vi "lowpass_derivative.vi"(9 "sigma_time":dbl=10.0 format="%#_13g", 10 "sampling frequency":dbl=0.1, 11 "X":dbl[](array[numeric])) -> (3 "dX":dbl[](array[numeric]))   [LabVIEW 2017]
uses:
  <vilib>/Analysis/2dsp.llb/1D Convolution (DBL).vi
  <vilib>/Analysis/1siggen.llb/General Gaussian Monopulse.vi
  <vilib>/Analysis/NI_AALBase.lvlib
  <vilib>/Analysis/NI_AALPro.lvlib
panel:
  out "input size":i32
  out "kernel size":i32
  out "Y":dbl[](graph)
  out "graph of dX":dbl[](graph)
  out "conv":dbl[](graph)
  out "X":dbl[](graph)
  out "pad size":i32
  out "conv size":i32
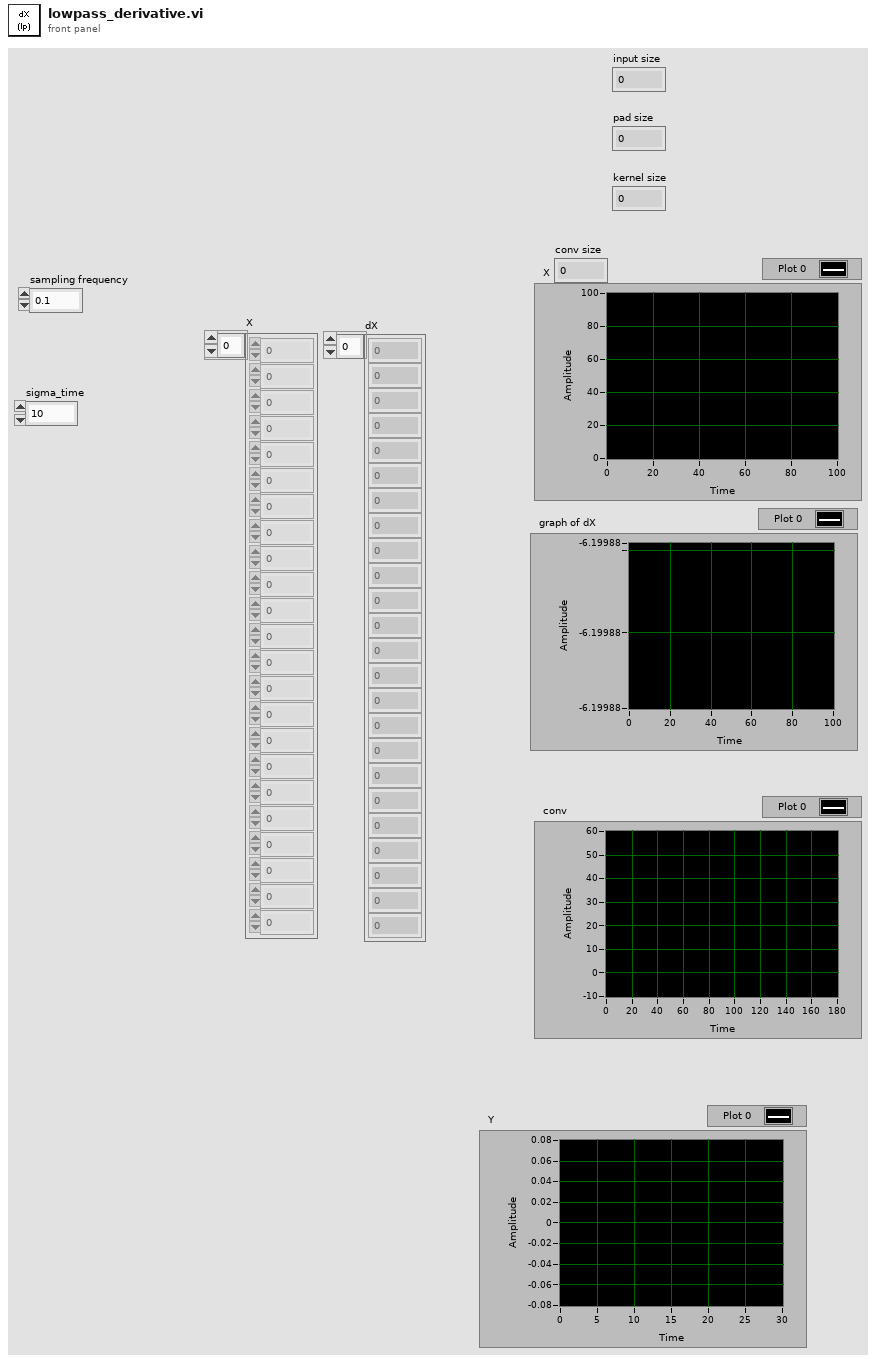
[diagram p1: front panel]
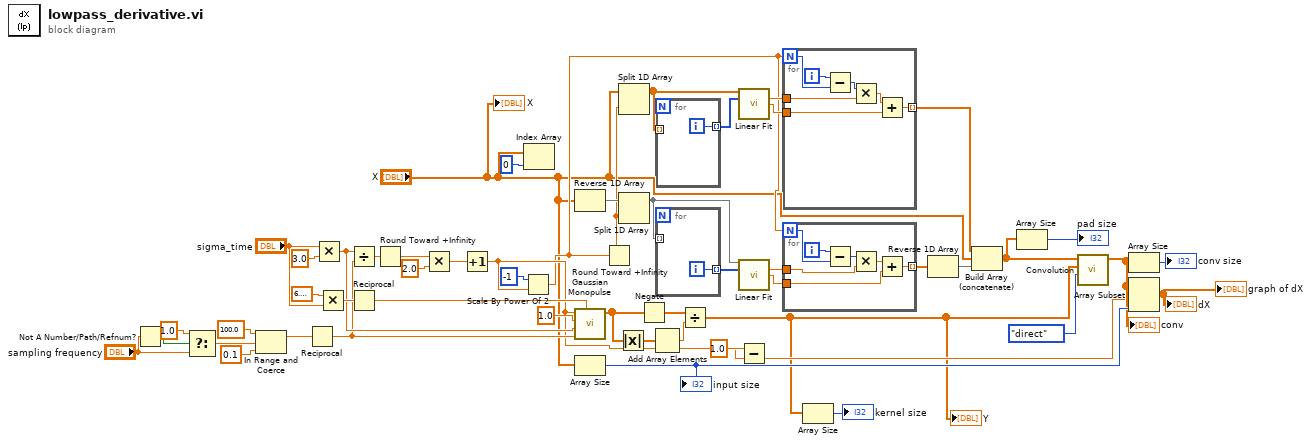
[diagram p0: block diagram]
diagram:
  n1 = Not A Number/Path/Refnum?(number/path/refnum="sampling frequency") -> (NaN/Path/Refnum?=w35:bool)
  n2 = Select(t=1.0, s=w35, f="sampling frequency") -> (s? t:f=w32:dbl)
  n3 = In Range and Coerce(upper limit=100.0, x=w32, lower limit=0.1) -> (coerced(x)=w38:dbl)  [unwired: 1 out]
  n4 = Reciprocal(x=w38) -> (1/x=w26:dbl)
  n5 = Multiply(x="sigma_time", y=3.0) -> (x*y=w47:dbl)
  n6 = Multiply(x=6.283185307179586, y="sigma_time") -> (x*y=w50:dbl)
  n7 = Divide(x=w47, y=w26) -> (x/y=w46:dbl)
  n8 = Reciprocal(x=w50) -> (1/x=w27:dbl)
  n9 = Round Toward +Infinity(x=w46) -> (ceil(x): smallest int >= x=w45:dbl)
  n10 = Multiply(x=w45, y=2.0) -> (x*y=w43:dbl)
  n11 = Increment(x=w43) -> (x+1=w8:dbl)
  n12 = Scale By Power Of 2(n=i16 -1, x=w8) -> (x*2^n=w3:dbl)
  n13 = Index Array(array="X", index=0) -> ()  [unwired: 1 out]
  n14 = Reverse 1D Array(array="X") -> (reversed array=w19:dbl[])
  n15 = call <vilib>:"Gaussian Monopulse.vi"("center frequency (Hz)"=w27, "delta t (s)"=w26, "delay (s)"=w47, "amplitude"=1.0, "samples"=w8) -> ("Gaussian Monopulse"=w28:dbl[])  [unwired: 5 in, 1 out]
  n16 = Array Size(array="X") -> (size(s)=w39:i32)
  "input size" <- w39
  n17 = Round Toward +Infinity(x=w3) -> (ceil(x): smallest int >= x=w16:dbl)
  n18 = Absolute Value(x=w28) -> (abs(x)=w41:dbl[])
  n19 = Split 1D Array(array="X", index=w16) -> (first subarray=w12:dbl[])  [unwired: 1 out]
  n20 = Split 1D Array(array=w19, index=w16) -> (first subarray=w15:dbl[])  [unwired: 1 out]
  n21 = Negate(x=w28) -> (-x=w2:dbl[])
  n22 = Add Array Elements(numeric array=w41) -> (sum=w25:dbl)
  n23 = for {
    tunnel: [w53] -> w24 mode=indexing
    tunnel: w12 -> [_] mode=indexing
    i -> [w53]
  }
  n24 = for {
    tunnel: [w54] -> w20 mode=indexing
    tunnel: w15 -> [_] mode=indexing
    i -> [w54]
  }
  n25 = Divide(x=w2, y=w25) -> (x/y=w5:dbl[])
  "Y" <- w5
  n26 = call <vilib>:"Linear Fit.vi"("Y"=w12, "X"=w24) -> ("slope"=w23:dbl, "intercept"=w22:dbl)  [unwired: 9 in, 3 out]
  n27 = call <vilib>:"Linear Fit.vi"("Y"=w15, "X"=w20) -> ("slope"=w18:dbl, "intercept"=w17:dbl)  [unwired: 9 in, 3 out]
  n28 = Subtract(x=w8, y=1.0 ("x")) -> (x-y=w7:dbl)
  n29 = for {
    N: w3 -> [w60]
    tunnel: w23 -> [w58]
    tunnel: w22 -> [w56]
    tunnel: [w55] -> w21 mode=indexing
    i -> [w61]
    n30 = Subtract(x=w61, y=w60) -> (x-y=w59:i32)
    n31 = Multiply(x=w59, y=w58) -> (x*y=w57:dbl)
    n32 = Add(x=w57, y=w56) -> (x+y=w55:dbl)
  }
  n33 = for {
    N: w3 -> [w67]
    tunnel: w18 -> [w65]
    tunnel: w17 -> [w63]
    tunnel: [w62] -> w14 mode=indexing
    i -> [w68]
    n34 = Subtract(x=w68, y=w67) -> (x-y=w66:i32)
    n35 = Multiply(x=w66, y=w65) -> (x*y=w64:dbl)
    n36 = Add(x=w64, y=w63) -> (x+y=w62:dbl)
  }
  n37 = Array Size(array=w5) -> (size(s)=→"kernel size":i32)
  n38 = Reverse 1D Array(array=w14) -> (reversed array=w13:dbl[])
  n39 = Build Array (concatenate)(w21, "X", w13) -> (w11:dbl[])
  n40 = Array Size(array=w11) -> (size(s)=→"pad size":i32)
  n41 = call-poly <vilib>:"Convolution.vi"("algorithm"=enum32{"direct", "frequency domain"}."direct", "Y"=w5, "X"=w11) -> ("X * Y"=w10:dbl[])  [unwired: 7 in, 1 out]
  "conv" <- w10
  n42 = Array Size(array=w10) -> (size(s)=→"conv size":i32)
  n43 = Array Subset(array=w10, index=w7, length=w39) -> (→"dX" →"graph of dX":dbl[])
  "X" <- "X"
